vi "test Get Base 16.vi"(11 "Test Case In":refnum<class "test EDS.lvclass">) -> (0 "error out":errorcluster, 3 "Test Case Out":refnum<class "test EDS.lvclass">)   [LabVIEW 2024, in "test EDS.lvclass"]
uses:
  test EDS.lvclass
  C:/Program Files/National Instruments/LabVIEW 2024/vi.lib/Astemes/LUnit/Test Case.lvclass
  <vilib>/Astemes/LUnit/Test Case.lvclass/Test Case.ctl
  <vilib>/Astemes/LUnit/Append Fail Result.vi
  <vilib>/Astemes/LUnit/Append Pass Result.vi
  <vilib>/Astemes/LUnit/Run In UI.vi
  <vilib>/Utility/error.llb/Clear Errors.vi
  Core/EDS.lvlib
  <vilib>/Astemes/LUnit/Test Case.lvclass
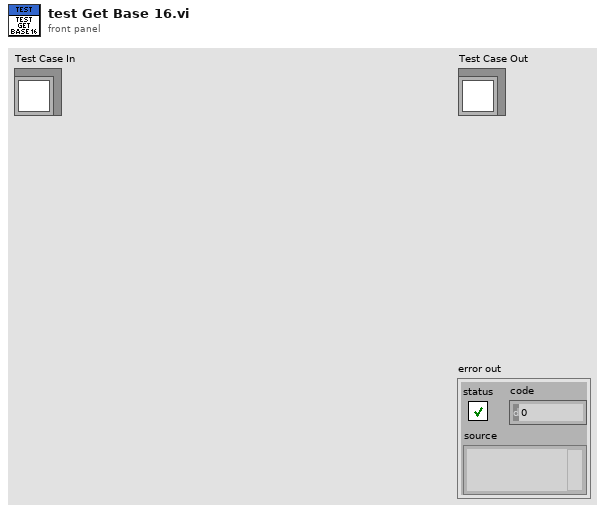
[diagram p1: front panel]
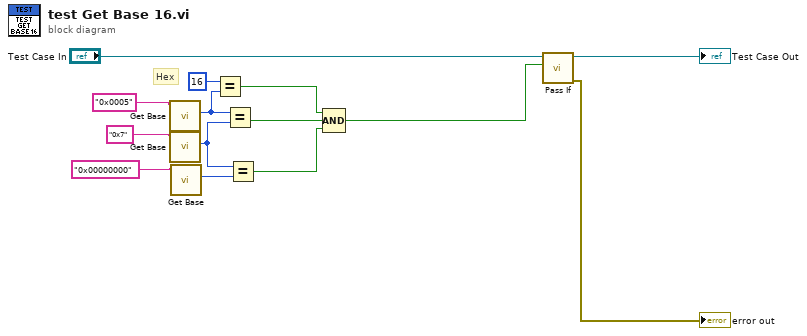
[diagram p0: block diagram]
diagram:
  # "Hex"
  n1 = call "Get Base.vi"("Default Value"="0x0005") -> ("Number Base"=w7:u8)  [unwired: 9 in, 1 out]
  n2 = call "Get Base.vi"("Default Value"="0x7") -> ("Number Base"=w5:u8)  [unwired: 9 in, 1 out]
  n3 = call "Get Base.vi"("Default Value"="0x00000000") -> ("Number Base"=w6:u8)  [unwired: 9 in, 1 out]
  n4 = Equal?(x=u8 16, y=w7) -> (x = y?=w4:bool)
  n5 = Equal?(x=w7, y=w5) -> (x = y?=w3:bool)
  n6 = Equal?(x=w5, y=w6) -> (x = y?=w2:bool)
  n7 = Compound Arithmetic op=AND(w4, w3, w2) -> (w1:bool)
  n8 = call <vilib>:"Pass If.vi"("Pass?"=w1, "LUnit Test Case In"="Test Case In") -> ("error out"=→"error out":errorcluster, "LUnit Test Case Out"=→"Test Case Out":refnum<class "test EDS.lvclass">)  [unwired: 8 in]
